vi "Create.vi"   [LabVIEW 2021, in "Field_RnD_Services_LIBSSH2_Toolkit.lvlib" / "Known Hosts.lvclass"]
doc: "Creates a new Known Hosts object that represents a libssh2lv shared library Known Hosts struct. This VI must be called, or executed, before using any other Known Hosts-related VIs. This VI allocates memory within the libssh2lv shared library that must be explicitly deallocated, or freed, at the end of the application using the <B>Destroy</B> VI to avoid memory leaks or running Out-of-Memory (OOM) on a resource contrained system.\n\nA Known Hosts object represents a linked list of entries in a known hosts file on the local host."
uses:
  220524-VNA RP FLAT.llb/Known Hosts.lvclass
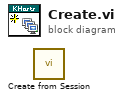
[diagram p0: block diagram]
diagram:
  n1 = call "Create from Session.vi"() -> ()  [unwired: 10 in, 2 out]
